vi "Register gRPC Parameters.vi"(8 "error in (no error)":errorcluster, 11 "OOP Server in":refnum<class "MeasurementService_Template.lvclass">) -> (0 "error out":errorcluster, 3 "OOP Server out":refnum<class "MeasurementService_Template.lvclass">)   [LabVIEW 2020, in "LoadRegulation.lvlib" / "MeasurementService_Template.lvclass"]
uses:
  MeasurementService_Template.lvclass
  MeasurementService_Template.lvclass/MeasurementService_Template.ctl
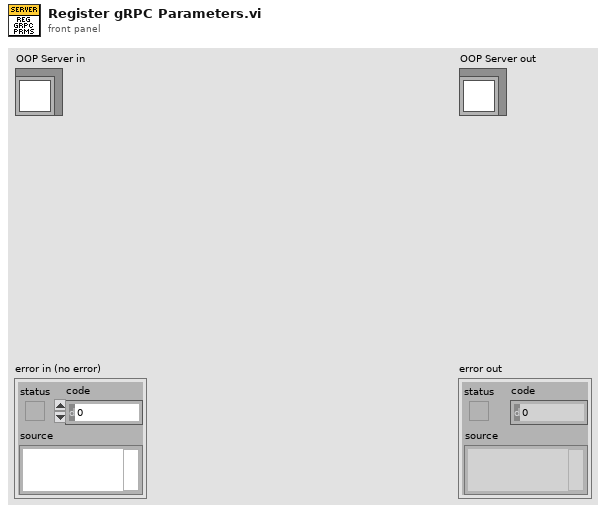
[diagram p1: front panel]
types:
  T1 = typedef "gprc-lvsupport-release.lvlib/grpcId.ctl" = u64
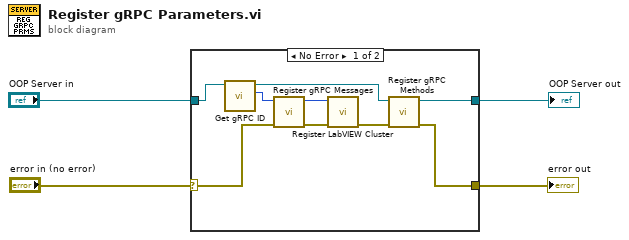
[diagram p0: block diagram]
diagram:
  n1 = case shown="No Error" "error in (no error)" {
    selector: "error in (no error)" -> [w13 w15]
    tunnel: [w12 w15] -> w3
    tunnel: [w8 w14] -> w1
    tunnel: "OOP Server in" -> [w11 w14]
    frame No Error {
      n2 = call "Get gRPC ID.vi"("OOP Server in"=w11) -> ("gRPC ID"=w10:T1, "OOP Server out"=w9:refnum<class "MeasurementService_Template.lvclass">)  [unwired: 9 in]
      n3 = call "Register gRPC Messages.vi"("error in (no error)"=w13, "gRPC ID"=w10) -> ("error out"=w6:errorcluster, "gRPC ID Out"=w7:T1)  [unwired: 8 in]
      n4 = call "Register LabVIEW Cluster.vi"("error in (no error)"=w6, "gRPC ID"=w7) -> ("error out"=w5:errorcluster)  [unwired: 8 in, 1 out]
      n5 = call "Register gRPC Methods.vi"("error in (no error)"=w5, "Template Server in"=w9) -> ("error out"=w12:errorcluster, "Template Server out"=w8:refnum<class "MeasurementService_Template.lvclass">)  [unwired: 8 in]
    }
    frame Error {
    }
  }
  "error out" <- w3
  "OOP Server out" <- w1
